vi "fucking PID -- V2.vi"(4 "PID parameters":T4={"I (sec)"=4.747474747474747, "P (sec)"=2.0765656565656565} {"P (sec)" scale=0.01..10.0; "I (sec)" scale=0.01..10.0}, 5 "dt (sec)":dbl=0.02 format="%#_10f", 6 "requested size":i32=100, 7 "PID action":T3, 8 "lorentzian IN":T1={"A (VHz)"=0.003914650866681924, "f (Hz)"=44855.11779996251, "G (Hz)"=2.9247633391664567, "phi(rad)"=3.909694945239435, "Q"=15336.32386569301, "Norm  Ampl"=nan, "bg (V)"=0.00013625172364348747-0.00019483842623467182i, "4corners"={"z (-pi/2)"=-0.0017563199699203156-0.00016210148449623068i, "z(inf)"=0.00013625172364348747-0.00019483842623467182i, "z (pi/2)"=0.0001689886653819286+0.0016977332673291314i, "z center"=-0.0007936656522691936+0.0007678158914164503i, "z(0)"=-0.0017235830281818747+0.0017304702090675725i, "radius"=0.0013384504702515796}} {"bg (V)" format="%#9_9f"; "Q" format="%#9_9f"; "phi(rad)" format="%#9_9f"; "G (Hz)" format="%#9_9f"; "f (Hz)" format="%#9_9f"}, 9 "voltage IN (V)":cdb=-0.0017981943418797428+0.0018232090265536353i format="%#_10f", 10 "time in (sec)":dbl=289.5873590533738, 11 "frequency IN (Hz)":dbl=-1.0 format="%#_10f") -> (0 "lorentzian  OUT":T1={"A (VHz)"=0.003914650866681924, "f (Hz)"=44855.11779996251, "G (Hz)"=2.9247633391664567, "phi(rad)"=3.909694945239435, "Q"=15336.32386569301, "Norm  Ampl"=nan, "bg (V)"=0.00013625172364348747-0.00019483842623467182i, "4corners"={"z (-pi/2)"=-0.0017563199699203156-0.00016210148449623068i, "z(inf)"=0.00013625172364348747-0.00019483842623467182i, "z (pi/2)"=0.0001689886653819286+0.0016977332673291314i, "z center"=-0.0007936656522691936+0.0007678158914164503i, "z(0)"=-0.0017235830281818747+0.0017304702090675725i, "radius"=0.0013384504702515796}} {"bg (V)" format="%#9_9f"; "Q" format="%#9_9f"; "phi(rad)" format="%#9_9f"; "G (Hz)" format="%#9_9f"; "f (Hz)" format="%#9_9f"}, 1 "v out":cdb[](array[numeric])=[-0.0018053953555071376+0.0018127409643177864i, -0.0018165156864968339+0.0018204053176322792i, -0.0017958469040712344+0.0018145950406335631i, -0.0018064864381374278+0.0018213989217676742i, -0.0018205836366976798+0.00181272131689436i, -0.0018068178418151558+0.0017978835138220595i, -0.0018112783584959197+0.0018131542902720791i, -0.001807623114856623+0.0018046251165330447i, -0.0018075769227948962+0.0018141191203122954i, -0.0018125924903436626+0.0018202640246869958i, -0.001797369769488581+0.0018281041177512854i, -0.001810807154127472+0.0018140671984214422i, -0.001801872080007094+0.0018103692059728753i, -0.0018200170226418007+0.0018069703355946354i, -0.0018044272125189902+0.0018419740527244371i, -0.0018048558055226668+0.0018054627086667766i, -0.0018000345238061355+0.001813547911683154i, -0.00179693547343068+0.001827074795896007i, -0.001816753685034828+0.0018283287859578406i, -0.0018100525624063777+0.0018375740151933535i, -0.0018020903561519347+0.001817810965243257i, -0.0018033487515777204+0.0018322759295837736i, -0.001812579170722185+0.0018085274657471593i, -0.0017986956233886219+0.0018369542975809256i, -0.0018110485423681176+0.0018179706114916812i, -0.001818585714895918+0.0018057011713030798i, -0.001817133445971395+0.0018057844840895796i, -0.001815295477436939+0.0018019924367636457i, -0.0018209260305803716+0.0018169201017635879i, -0.0018044295722803938+0.0018022115018756124i, -0.0018311116336601925+0.0018193183868968638i, -0.0018101122757938476+0.0018192759665263973i, -0.0018085434485789354+0.0018163840717862938i, -0.001811836070789227+0.0018293939486975547i, -0.0018092170283701484+0.0018335734859818993i, -0.0018027628167522247+0.0018175751194074211i, -0.0018166463462358528+0.0018270586309948938i, -0.0018043289950367871+0.0018167107559412144i, -0.0018133661975601213+0.0018067609986972299i, -0.0017964121526070878+0.0018212577751918577i, -0.0018005011585912297+0.0018307733988123496i, -0.0018055089150084513+0.0018207057552428135i, -0.0017933683638453196+0.0018290393276094053i, -0.0017947337607063093+0.0018293596839623776i, -0.0018050366985486908+0.0018131516359867486i, -0.001823410598729327+0.0018322386017997551i, -0.0018213270704244217+0.0018092401922307647i, -0.0018195368344010806+0.0018317652375891755i, -0.0018122690298869983+0.0018107874585092214i, -0.0018117815927876852+0.0018193417970865829i, -0.0018241277734167283+0.0018110267815123905i, -0.0018134767100775348+0.0017996041850788186i, -0.0018085781667024604+0.0018109931540198922i, -0.001812588195649308+0.0018242546775294286i, -0.0018038342733790107+0.001816579416119673i, -0.0018219581923603048+0.0018186401375626616i, -0.0018082074467579577+0.0018250013278144528i, -0.0018010302913536497+0.0018340252731910817i, -0.0018095892512791758+0.0018082746963879737i, -0.001806173137863751+0.0018278464093150928i, -0.001806209423211567+0.0018248931786284301i, -0.0018050281395048705+0.0018214527143317128i, -0.001813147159223057+0.0018166873546764629i, -0.0018195040297905845+0.0018213362095911285i, -0.0018038880195332188+0.0018363883332626796i, -0.001811734461819379+0.0018334572150754632i, -0.0018197474636337785+0.001827200887836666i, -0.0017993690496703942+0.0018175740841111926i, -0.0018013879772756337+0.0018034726194164816i, -0.0018044338062849698+0.0018054946939652574i, -0.0018069258232117898+0.001804782758233771i, -0.0018053566300732108+0.001813146961088779i, -0.0018108387556523507+0.0018223068444301986i, -0.0018055103162283466+0.0018170190046832937i, -0.001796024867922929+0.0018240437769777192i, -0.00181063889885541+0.0018058095935931078i, -0.001816760169916204+0.0018115543327705717i, -0.001821094189462785+0.0018078193998815753i, -0.0018114690511362443+0.0018162294699294935i, -0.0018205201141340865+0.001815460678585127i, -0.0017960813076323245+0.0018219635616207451i, -0.0018133234755257535+0.001825049411969287i, -0.001793713870756671+0.001828469705839483i, -0.0018197224487349053+0.001820094212900604i, -0.0018034364661581844+0.0018195335089581947i, -0.0018117189448709056+0.0018188356639653775i, -0.0018008807106835575+0.0018082984011016196i, -0.001802397549962857+0.0018234420699496804i, -0.0018020531158325977+0.0018153058250442436i, -0.0018119913919984066+0.0018153898036333176i, -0.0018073563404384567+0.001819477319147889i, -0.0018121809440278865+0.0018111441608997885i, -0.0018242548595987654+0.0018095956861807342i, -0.0018181047305480982+0.0018060237749628657i, -0.0018154249912101326+0.001810587721306845i, -0.0018155727208419678+0.0018124932447052052i, -0.0018045211817166694+0.0018251170721478073i, -0.0017910521384331079+0.0018331825634809928i, -0.0018064879357469722+0.00182378857110241i, -0.0017981943418797428+0.0018232090265536353i], 2 "freq out":dbl[](array[numeric])=[44853.954031385074, 44853.95417850819, 44853.95416410566, 44853.95436984526, 44853.954673103784, 44853.95452102071, 44853.95394456051, 44853.95323936248, 44853.95230715085, 44853.95139559195, 44853.95052494639, 44853.95024214874, 44853.94983252503, 44853.949439049786, 44853.94854203172, 44853.94838555576, 44853.948031097505, 44853.94780607535, 44853.94808777986, 44853.9483726385, 44853.94903629037, 44853.9497722594, 44853.950879112366, 44853.9515405353, 44853.9528019089, 44853.9538597573, 44853.95426613575, 44853.95412636491, 44853.95345285364, 44853.952516460304, 44853.95139778942, 44853.94987487855, 44853.948493955875, 44853.94721042105, 44853.94623774795, 44853.94570350666, 44853.94534559761, 44853.94503106676, 44853.94481159447, 44853.94422572135, 44853.94406163855, 44853.94439703849, 44853.94482391797, 44853.94582142724, 44853.94730382804, 44853.948592177054, 44853.94970877772, 44853.95018506272, 44853.95065691107, 44853.95081055912, 44853.95089133452, 44853.95041517962, 44853.94942821411, 44853.948370230835, 44853.94746170018, 44853.946719537955, 44853.945737128226, 44853.94501943662, 44853.944922088354, 44853.94457202579, 44853.94453569174, 44853.94471054988, 44853.94502285759, 44853.94515064288, 44853.94506873293, 44853.94552585551, 44853.94620773221, 44853.94675248255, 44853.94744256621, 44853.94788303192, 44853.94807376572, 44853.94796538342, 44853.94782032052, 44853.94772674184, 44853.94768361845, 44853.94807950944, 44853.94808782982, 44853.94773645385, 44853.9468712699, 44853.94597506698, 44853.94481511086, 44853.94416172561, 44853.94361605697, 44853.94372148111, 44853.943585372836, 44853.943613136726, 44853.94357093545, 44853.943481781476, 44853.94366789763, 44853.94391882446, 44853.94398923662, 44853.944105616014, 44853.943951605856, 44853.943228697484, 44853.94206051962, 44853.94066552022, 44853.93910863893, 44853.93796875516, 44853.93771672214, 44853.93766607227], 3 "frequency out (Hz)":dbl=44853.937983312026 format="%#_10f")   [LabVIEW 2018]
uses:
  pid -- parameters.ctl
  PID action.ctl
  lorentzian.ctl
  circle corners.ctl
  four-corner circle transformation.ctl
  agregator -- action.ctl
  linear interpolation iiii- complex.vi
  linear interpolation - real.vi
  Q - not nan -- real.vi
panel:
  out "Plot: complex plane":cluster{dbl[], dbl[]}[](graph)=[{[], []}, {[nan, nan, nan, nan, nan, nan, nan, nan, nan, nan, nan, nan, nan, nan, nan, nan, nan, nan, nan, nan, nan, nan, nan, nan, nan, nan, nan, nan, nan, nan, nan, nan, nan, nan, nan, nan, nan, nan, nan, nan, nan, nan, nan, nan, nan, nan, nan, nan, nan, nan], [nan, nan, nan, nan, nan, nan, nan, nan, nan, nan, nan, nan, nan, nan, nan, nan, nan, nan, nan, nan, nan, nan, nan, nan, nan, nan, nan, nan, nan, nan, nan, nan, nan, nan, nan, nan, nan, nan, nan, nan, nan, nan, nan, nan, nan, nan, nan, nan, nan, nan]}, {[nan, nan, nan, nan, nan, nan, nan, nan, nan, nan, nan, nan, nan, nan, nan, nan, nan, nan, nan, nan], [nan, nan, nan, nan, nan, nan, nan, nan, nan, nan, nan, nan, nan, nan, nan, nan, nan, nan, nan, nan]}, {[nan, nan, nan, nan, nan, nan, nan, nan, nan, nan, nan, nan, nan, nan, nan, nan, nan, nan, nan, nan], [nan, nan, nan, nan, nan, nan, nan, nan, nan, nan, nan, nan, nan, nan, nan, nan, nan, nan, nan, nan]}, {[nan, nan, nan, nan, nan, nan, nan, nan, nan, nan, nan, nan, nan, nan, nan, nan, nan, nan, nan, nan], [nan, nan, nan, nan, nan, nan, nan, nan, nan, nan, nan, nan, nan, nan, nan, nan, nan, nan, nan, nan]}, {[nan, nan, nan, nan, nan, nan, nan, nan, nan, nan, nan, nan, nan, nan, nan, nan, nan, nan, nan, nan], [nan, nan, nan, nan, nan, nan, nan, nan, nan, nan, nan, nan, nan, nan, nan, nan, nan, nan, nan, nan]}, {[], []}]
  in  "Plot: complex plane - filter":cluster{dbl[], dbl[]}[](graph)=[{[], []}, {[], []}, {[0.0, 0.0, 0.0, 0.0, 0.0, 0.0, 0.0, 0.0, 0.0, 0.0, 0.0, 0.0, 0.0, 0.0, 0.0, 0.0, 0.0, 0.0, 0.0, 0.0, 0.0, 0.0, 0.0, 0.0, 0.0, 0.0, 0.0, 0.0, 0.0, 0.0, 0.0, 0.0, 0.0, 0.0, 0.0, 0.0, 0.0, 0.0, 0.0, 0.0, 0.0, 0.0, 0.0, 0.0, 0.0, 0.0, 0.0, 0.0, 0.0, 0.0, 0.0, 0.0, 0.0, 0.0, 0.0, 0.0, 0.0, 0.0, 0.0, 0.0, 0.0, 0.0, 0.0, 0.0, 0.0, 0.0, 0.0, 0.0, 0.0, 0.0, 0.0, 0.0, 0.0, 0.0, 0.0, 0.0, 0.0, 0.0, 0.0, 0.0, 0.0, 0.0, 0.0, 0.0, 0.0, 0.0, 0.0, 0.0, 0.0, 0.0, 0.0, 0.0, 0.0, 0.0, 0.0, 0.0, 0.0, 0.0, 0.0, 0.0], [0.0, 0.0, 0.0, 0.0, 0.0, 0.0, 0.0, 0.0, 0.0, 0.0, 0.0, 0.0, 0.0, 0.0, 0.0, 0.0, 0.0, 0.0, 0.0, 0.0, 0.0, 0.0, 0.0, 0.0, 0.0, 0.0, 0.0, 0.0, 0.0, 0.0, 0.0, 0.0, 0.0, 0.0, 0.0, 0.0, 0.0, 0.0, 0.0, 0.0, 0.0, 0.0, 0.0, 0.0, 0.0, 0.0, 0.0, 0.0, 0.0, 0.0, 0.0, 0.0, 0.0, 0.0, 0.0, 0.0, 0.0, 0.0, 0.0, 0.0, 0.0, 0.0, 0.0, 0.0, 0.0, 0.0, 0.0, 0.0, 0.0, 0.0, 0.0, 0.0, 0.0, 0.0, 0.0, 0.0, 0.0, 0.0, 0.0, 0.0, 0.0, 0.0, 0.0, 0.0, 0.0, 0.0, 0.0, 0.0, 0.0, 0.0, 0.0, 0.0, 0.0, 0.0, 0.0, 0.0, 0.0, 0.0, 0.0, 0.0]}, {[0.0, 0.0, 0.0], [0.0, 0.0, 0.0]}, {[nan, nan, nan, nan, nan, nan, nan, nan, nan, nan, nan, nan, nan, nan, nan, nan, nan, nan, nan, nan], [nan, nan, nan, nan, nan, nan, nan, nan, nan, nan, nan, nan, nan, nan, nan, nan, nan, nan, nan, nan]}, {[0.0, 0.0, 0.0, 0.0, 0.0, 0.0, 0.0, 0.0, 0.0, 0.0, 0.0, 0.0, 0.0, 0.0, 0.0, 0.0, 0.0, 0.0, 0.0, 0.0], [0.0, 0.0, 0.0, 0.0, 0.0, 0.0, 0.0, 0.0, 0.0, 0.0, 0.0, 0.0, 0.0, 0.0, 0.0, 0.0, 0.0, 0.0, 0.0, 0.0]}]
  out "pm lorentzian":T1={"A (VHz)"=nan, "f (Hz)"=0.0, "G (Hz)"=0.0, "phi(rad)"=nan, "Q"=nan, "Norm  Ampl"=nan, "bg (V)"=nan+nani, "4corners"={"z (-pi/2)"=nan+nani, "z(inf)"=nan+nani, "z (pi/2)"=nan+nani, "z center"=nan+nani, "z(0)"=nan+nani, "radius"=nan}} {"bg (V)" format="%#9_9f"; "Q" format="%#9_9f"; "phi(rad)" format="%#9_9f"; "G (Hz)" format="%#9_9f"; "f (Hz)" format="%#9_9f"}
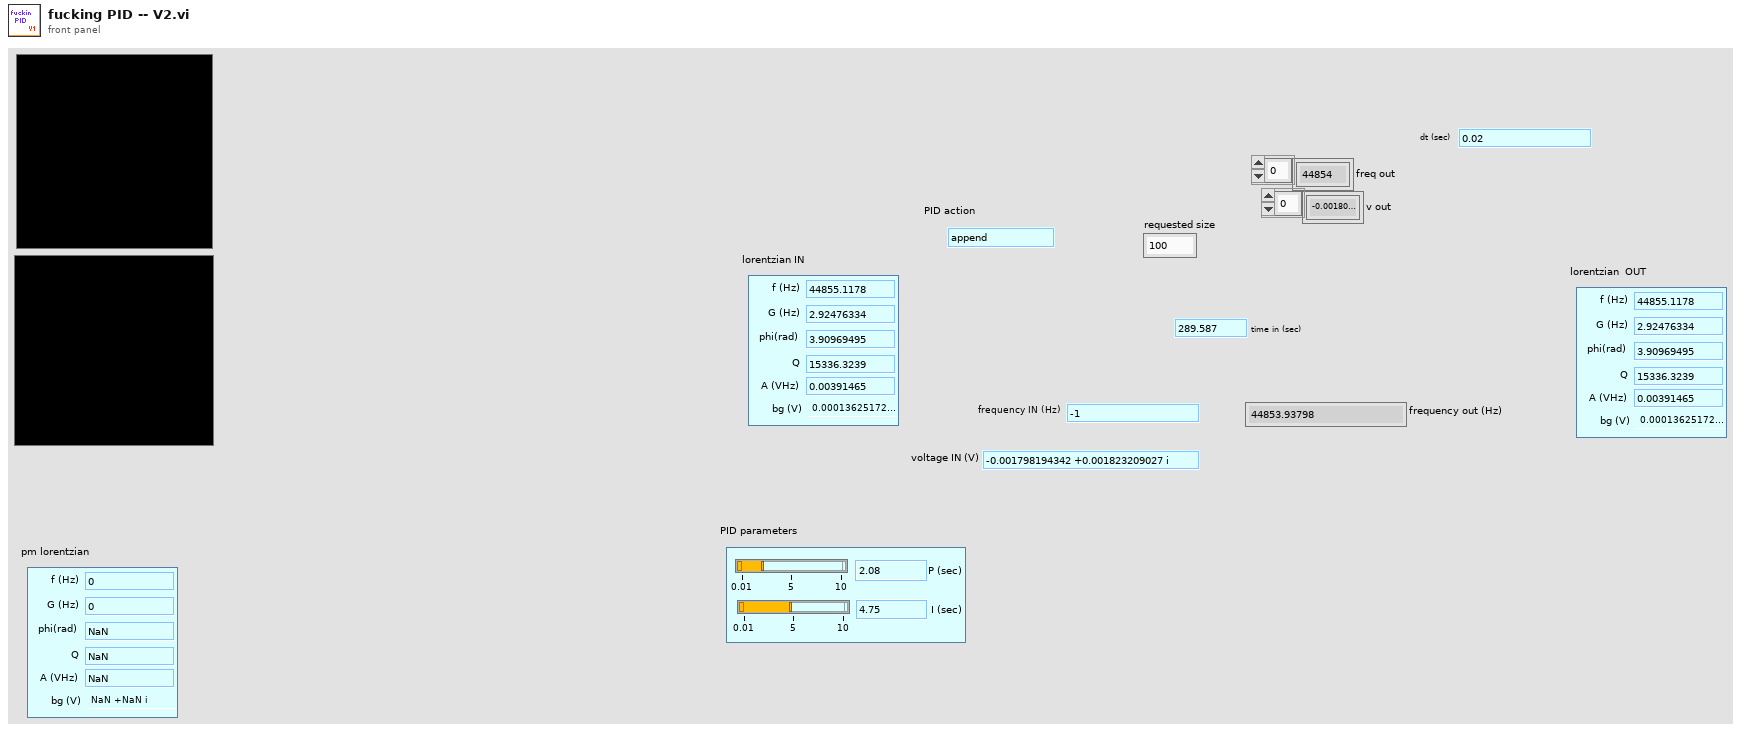
[diagram p1: front panel]
types:
  T1 = typedef "lorentzian.ctl" = cluster{"A (VHz)":dbl, "f (Hz)":dbl, "G (Hz)":dbl, "phi(rad)":dbl, "Q":dbl, "Norm  Ampl":dbl, "bg (V)":cdb, "4corners":T2}
  T2 = typedef "circle corners.ctl" = cluster{"z (-pi/2)":cdb, "z(inf)":cdb, "z (pi/2)":cdb, "z center":cdb, "z(0)":cdb, "radius":dbl}
  T3 = typedef "PID action.ctl" = enum16{"append", "empty!", "reset frequency", "reset from num", "overlimit"}
  T4 = typedef "pid -- parameters.ctl" = cluster{"I (sec)":dbl, "P (sec)":dbl}
  T5 = typedef "four-corner circle transformation.ctl" = enum16{"z(c) z(inf)", "z(c) z(zero)", "fix phase", "calculate lorentzian", "z(0) z(+-pi/2)", "shift to zcenter", "to  canonical", "get canonical phase", "get4corners", "update lorentzian -- from z0", "fake gamma normal", "fake gamma heat", "calculate complex slope"}
  T6 = typedef "agregator -- action.ctl" = enum16{"append", "interpolate", "empty!", "force", "init", "scale", "read last"}
  T7 = typedef "interpolation state - real.ctl" = cluster{"requested size":i32, "Array":dbl[], "actual number of elements":i32}
  T8 = typedef "interpolation state - complex.ctl" = cluster{"requested size":i32, "Array":cdb[], "actual number of elements":i32}
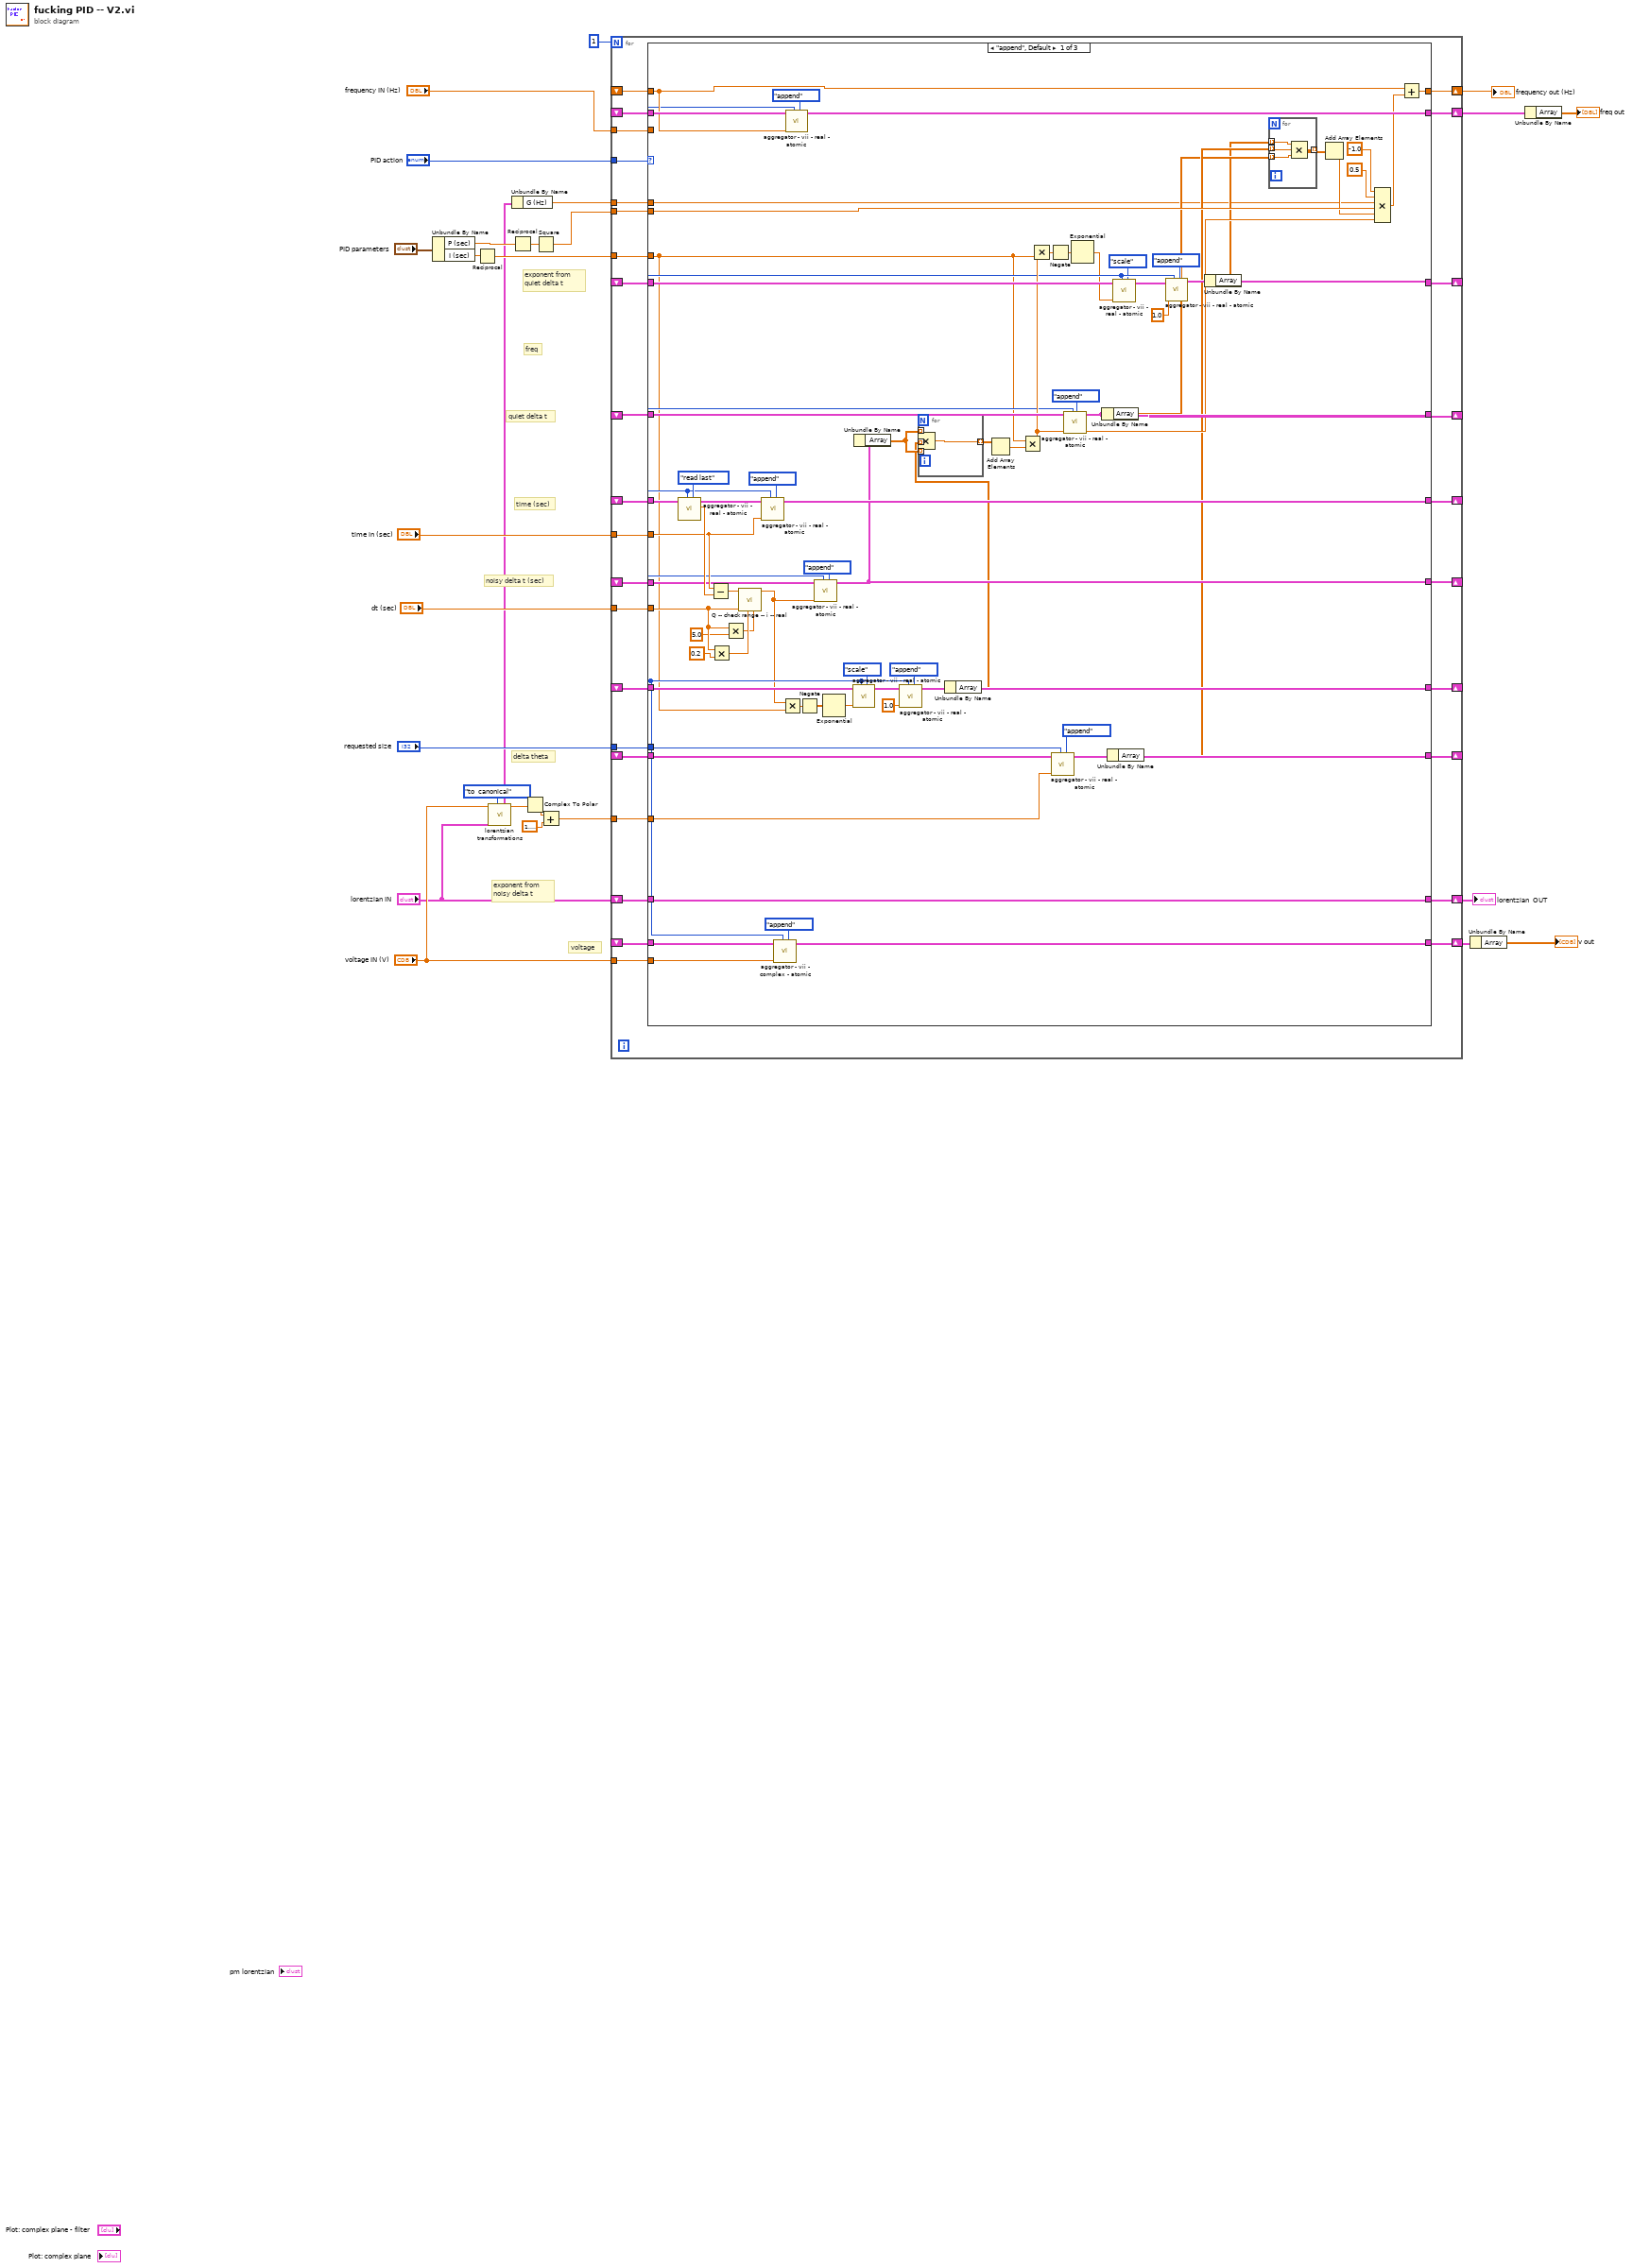
[diagram p0: block diagram]
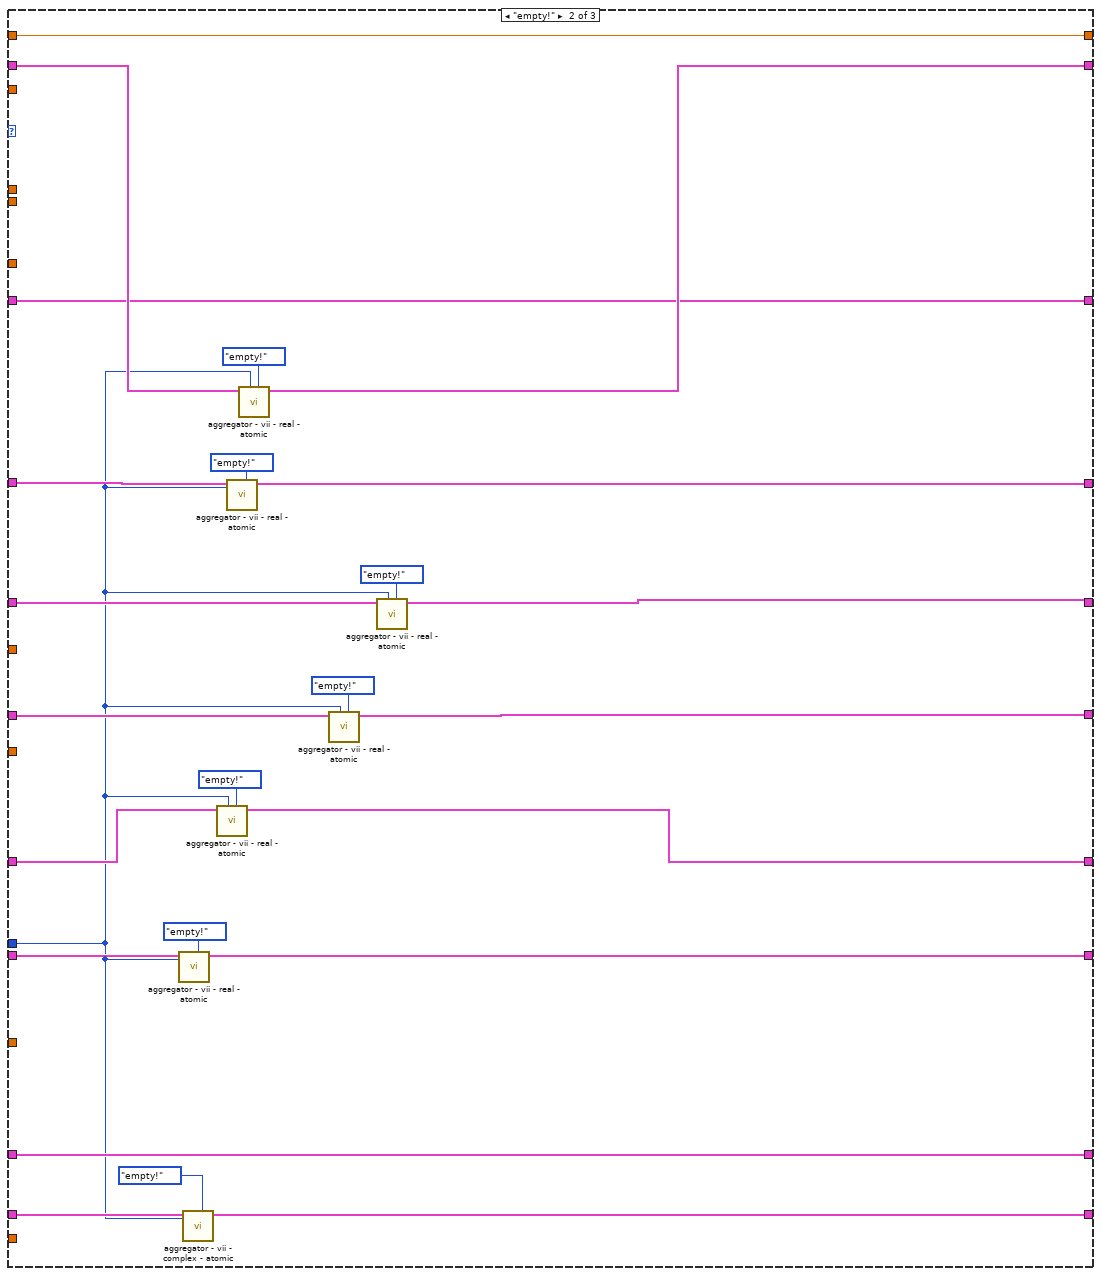
[diagram p2: hidden frame]
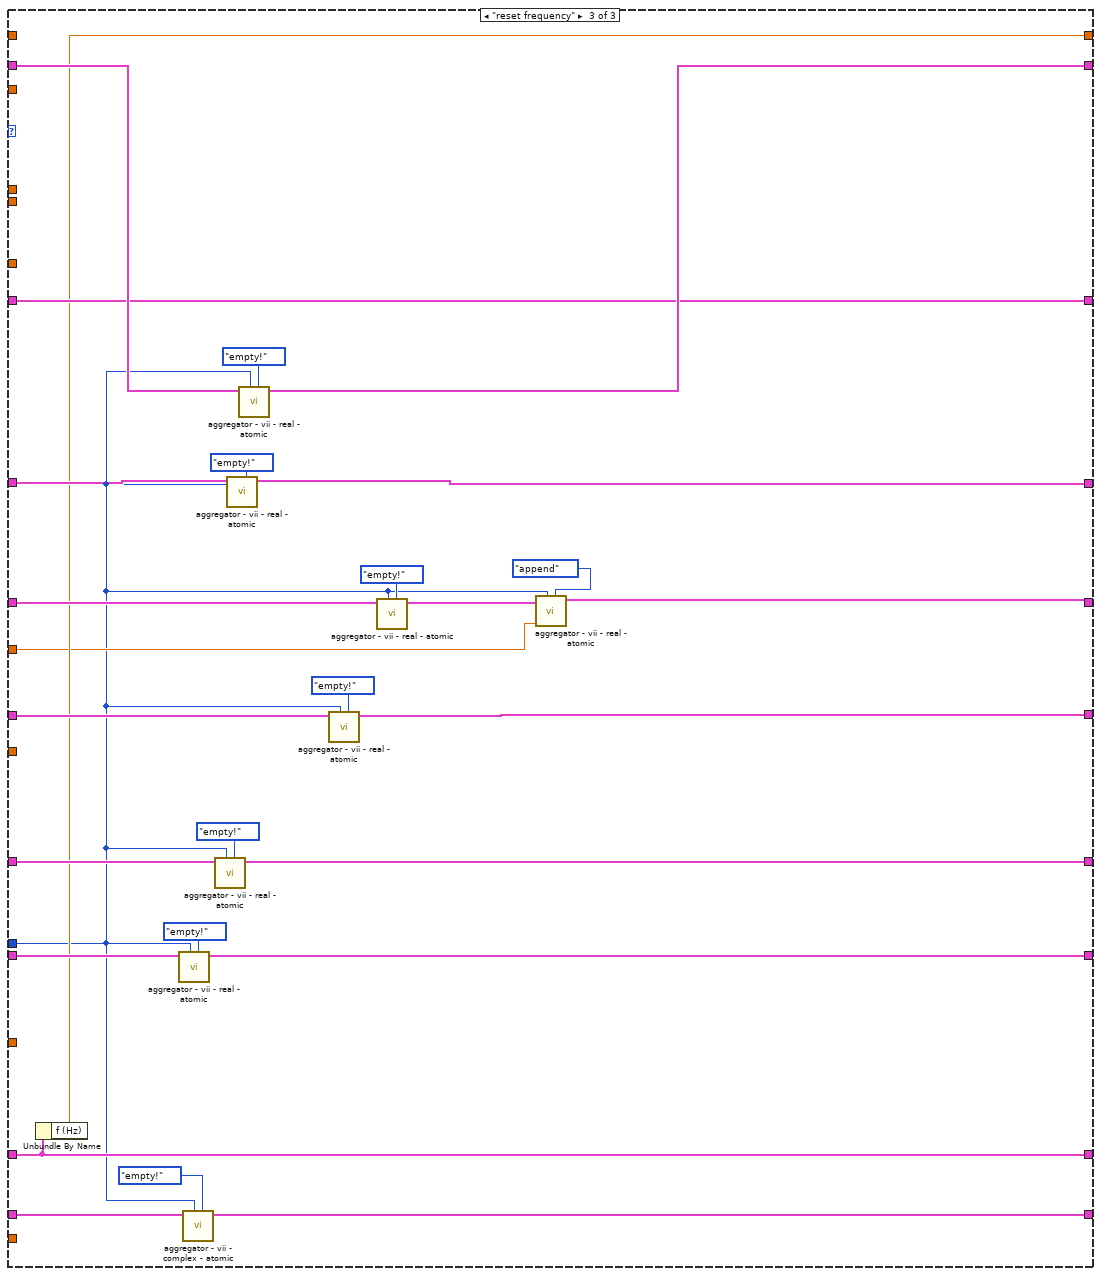
[diagram p3: hidden frame]
diagram:
  # "voltage"
  # "freq"
  # "delta theta"
  # "exponent from \nquiet delta t"
  # "quiet delta t"
  # "time (sec)"
  # "noisy delta t (sec)"
  # "exponent from \nnoisy delta t"
  n1 = Unbundle By Name("PID parameters") -> ("P (sec)"=w19:dbl, "I (sec)"=w21:dbl)
  n2 = Reciprocal(x=w21) -> (1/x=w20:dbl)
  n3 = call "lorentzian transformations.vi"("4 corner circle transformation"=four-corner_circle_transformation."to  canonical", "lorentzian in"="lorentzian IN", "voltage in"="voltage IN (V)") -> ("voltage out"=w7:cdb)  [unwired: 5 in, 3 out]
  n4 = Unbundle By Name("lorentzian IN") -> ("G (Hz)"=w2:dbl)
  n5 = Reciprocal(x=w19) -> (1/x=w18:dbl)
  n6 = Complex To Polar(r * e^(i*theta)=w7) -> (theta=w8:dbl)  [unwired: 1 out]
  n7 = Square(x=w18) -> (x^2=w17:dbl)
  n8 = Add(x=w8, y=1.5707963267948966) -> (x+y=w3:dbl)
  n9 = for {
    N: 1 -> [_]
    tunnel: "requested size" -> [w56]
    tunnel: "PID action" -> [w55]
    shift-right: [w53] -> _
    shift-left: _ -> [w54]
    tunnel: "time in (sec)" -> [w52]
    shift-right: [w50] -> _
    shift-left: _ -> [w51]
    tunnel: w20 -> [w49]
    tunnel: "voltage IN (V)" -> [w48]
    shift-right: [w46] -> _
    shift-left: _ -> [w47]
    shift-right: [w44] -> _
    shift-left: _ -> [w45]
    tunnel: w17 -> [w42]
    shift-right: [w41] -> w16
    shift-left: _ -> [w43]
    shift-right: [w40] -> w15
    shift-left: "lorentzian IN" -> [w39]
    shift-right: [w38] -> w12
    shift-left: _ -> [w37]
    shift-right: [w36] -> w14
    shift-left: _ -> [w35]
    shift-right: [w34] -> _
    shift-left: _ -> [w33]
    shift-right: [w32] -> _
    shift-left: _ -> [w31]
    tunnel: "frequency IN (Hz)" -> [w30]
    tunnel: "dt (sec)" -> [w29]
    tunnel: w3 -> [w28]
    tunnel: w2 -> [w27]
    n10 = case shown="\"append\", Default" w55 {
      tunnel: w56 -> [w83 w135 w159]
      tunnel: w54 -> [w125 w148 w176]
      tunnel: [w105 w134 w161] -> w53
      tunnel: w52 -> [w116 _ w160]
      tunnel: w51 -> [w124 w152 w180]
      tunnel: [w110 w151 w179] -> w50
      tunnel: w49 -> [w62 _ _]
      tunnel: w48 -> [w99 _ _]
      tunnel: w47 -> [w91 w150 w178]
      tunnel: [w78 w149 w177] -> w46
      tunnel: w45 -> [w114 w154 w182]
      tunnel: [w112 w153 w181] -> w44
      tunnel: w43 -> [w96 w147 _]
      tunnel: w39 -> [w102 w146 w165]
      tunnel: w42 -> [w109 _ _]
      tunnel: [w107 w147 w164] -> w41
      tunnel: [w102 w146 w165] -> w40
      tunnel: [w101 w144 w174] -> w38
      tunnel: w37 -> [w100 w145 w175]
      tunnel: [w98 w140 w170] -> w36
      tunnel: w35 -> [w97 w141 w171]
      tunnel: [w80 w138 w168] -> w34
      tunnel: w33 -> [w88 w137 w167]
      tunnel: [w79 w136 w166] -> w32
      tunnel: w31 -> [w87 w136 w166]
      tunnel: w30 -> [_ _ _]
      tunnel: w29 -> [w63 _ _]
      tunnel: w28 -> [w58 _ _]
      tunnel: w27 -> [w57 _ _]
      frame "append", Default {
        n11 = call "aggregator - vii - real - atomic.vi"("aggregator action"=agregator_--_action."read last", "requested size"=w83, "state IN"=w125) -> ("mean"=w118:dbl, "state OUT"=w106:T7)  [unwired: 5 in, 2 out]
        n12 = Subtract(x=w116, y=w118) -> (x-y=w73:dbl)
        n13 = Multiply(x=w63, y=0.2 ("upper")) -> (x*y=w69:dbl)
        n14 = Multiply(x=w63, y=5.0 ("upper")) -> (x*y=w60:dbl)
        n15 = call "Q -- check range -- i -- real.vi"("upper"=w60, "lower"=w69, "default"=w63, "number"=w73) -> ("number in range"=w71:dbl)  [unwired: 5 in, 2 out]
        n16 = call "aggregator - vii - real - atomic.vi"("aggregator action"=agregator_--_action."append", "requested size"=w83, "number"=w116, "state IN"=w106) -> ("state OUT"=w105:T7)  [unwired: 4 in, 3 out]
        n17 = call "aggregator - vii - complex - atomic.vi"("aggregator action"=agregator_--_action."append", "requested size"=w83, "number"=w99, "state IN"=w100) -> ("state OUT"=w101:T8)  [unwired: 4 in, 3 out]
        n18 = Multiply(x=w71, y=w62) -> (x*y=w75:dbl)
        n19 = call "aggregator - vii - real - atomic.vi"("aggregator action"=agregator_--_action."append", "requested size"=w83, "number"=w96, "state IN"=w97) -> ("state OUT"=w98:T7)  [unwired: 4 in, 3 out]
        n20 = Negate(x=w75) -> (-x=w72:dbl)
        n21 = call "aggregator - vii - real - atomic.vi"("aggregator action"=agregator_--_action."append", "requested size"=w83, "number"=w71, "state IN"=w91) -> ("state OUT"=w78:T7)  [unwired: 4 in, 3 out]
        n22 = Exponential(1:w72) -> (0:w74:dbl)
        n23 = call "aggregator - vii - real - atomic.vi"("aggregator action"=agregator_--_action."scale", "requested size"=w83, "number"=w74, "state IN"=w124) -> ("state OUT"=w123:T7)  [unwired: 4 in, 3 out]
        n24 = Unbundle By Name(w78) -> ("Array"=w90:dbl[])
        n25 = call "aggregator - vii - real - atomic.vi"("aggregator action"=agregator_--_action."append", "requested size"=w83, "number"=1.0, "state IN"=w123) -> ("state OUT"=w110:T7)  [unwired: 4 in, 3 out]
        n26 = Unbundle By Name(w110) -> ("Array"=w77:dbl[])
        n27 = for {
          tunnel: [w129] -> w92 mode=indexing
          tunnel: w90 -> [w128] mode=indexing
          tunnel: w77 -> [w127] mode=indexing
          tunnel: w90 -> [w126] mode=indexing
          n28 = Compound Arithmetic op=MULTIPLY(w128, w127, w126) -> (w129:dbl)
        }
        n29 = Add Array Elements(numeric array=w92) -> (sum=w61:dbl)
        n30 = Multiply(x=w62, y=w61) -> (x*y=w86:dbl)
        n31 = Multiply(x=w86, y=w62) -> (x*y=w66:dbl)
        n32 = Negate(x=w66) -> (-x=w65:dbl)
        n33 = call "aggregator - vii - real - atomic.vi"("aggregator action"=agregator_--_action."append", "requested size"=w83, "number"=w58, "state IN"=w114) -> ("state OUT"=w112:T7)  [unwired: 4 in, 3 out]
        n34 = call "aggregator - vii - real - atomic.vi"("aggregator action"=agregator_--_action."append", "requested size"=w83, "number"=w86, "state IN"=w88) -> ("state OUT"=w80:T7)  [unwired: 4 in, 3 out]
        n35 = Exponential(1:w65) -> (0:w64:dbl)
        n36 = Unbundle By Name(w80) -> ("Array"=w68:dbl[])
        n37 = Unbundle By Name(w112) -> ("Array"=w76:dbl[])
        n38 = call "aggregator - vii - real - atomic.vi"("aggregator action"=agregator_--_action."scale", "requested size"=w83, "number"=w64, "state IN"=w87) -> ("state OUT"=w85:T7)  [unwired: 4 in, 3 out]
        n39 = call "aggregator - vii - real - atomic.vi"("aggregator action"=agregator_--_action."append", "requested size"=w83, "number"=1.0, "state IN"=w85) -> ("state OUT"=w79:T7)  [unwired: 4 in, 3 out]
        n40 = Unbundle By Name(w79) -> ("Array"=w67:dbl[])
        n41 = for {
          tunnel: w76 -> [w133] mode=indexing
          tunnel: [w132] -> w111 mode=indexing
          tunnel: w68 -> [w131] mode=indexing
          tunnel: w67 -> [w130] mode=indexing
          n42 = Compound Arithmetic op=MULTIPLY(w130, w133, w131) -> (w132:dbl)
        }
        n43 = Add Array Elements(numeric array=w111) -> (sum=w108:dbl)
        n44 = Compound Arithmetic op=MULTIPLY(-1.0 ("value"), 0.5 ("value"), w57, w109, w108, w86) -> (w93:dbl)
        n45 = Add(x=w96, y=w93) -> (x+y=w107:dbl)
      }
      frame "empty!" {
        n46 = call "aggregator - vii - real - atomic.vi"("aggregator action"=agregator_--_action."empty!", "requested size"=w135, "state IN"=w154) -> ("state OUT"=w153:T7)  [unwired: 5 in, 3 out]
        n47 = call "aggregator - vii - complex - atomic.vi"("aggregator action"=agregator_--_action."empty!", "requested size"=w135, "state IN"=w145) -> ("state OUT"=w144:T8)  [unwired: 5 in, 3 out]
        n48 = call "aggregator - vii - real - atomic.vi"("aggregator action"=agregator_--_action."empty!", "requested size"=w135, "state IN"=w152) -> ("state OUT"=w151:T7)  [unwired: 5 in, 3 out]
        n49 = call "aggregator - vii - real - atomic.vi"("aggregator action"=agregator_--_action."empty!", "requested size"=w135, "state IN"=w137) -> ("state OUT"=w138:T7)  [unwired: 5 in, 3 out]
        n50 = call "aggregator - vii - real - atomic.vi"("aggregator action"=agregator_--_action."empty!", "requested size"=w135, "state IN"=w141) -> ("state OUT"=w140:T7)  [unwired: 5 in, 3 out]
        n51 = call "aggregator - vii - real - atomic.vi"("aggregator action"=agregator_--_action."empty!", "requested size"=w135, "state IN"=w150) -> ("state OUT"=w149:T7)  [unwired: 5 in, 3 out]
        n52 = call "aggregator - vii - real - atomic.vi"("aggregator action"=agregator_--_action."empty!", "requested size"=w135, "state IN"=w148) -> ("state OUT"=w134:T7)  [unwired: 5 in, 3 out]
      }
      frame "reset frequency" {
        n53 = Unbundle By Name(w165) -> ("f (Hz)"=w164:dbl)
        n54 = call "aggregator - vii - real - atomic.vi"("aggregator action"=agregator_--_action."empty!", "requested size"=w159, "state IN"=w182) -> ("state OUT"=w181:T7)  [unwired: 5 in, 3 out]
        n55 = call "aggregator - vii - complex - atomic.vi"("aggregator action"=agregator_--_action."empty!", "requested size"=w159, "state IN"=w175) -> ("state OUT"=w174:T8)  [unwired: 5 in, 3 out]
        n56 = call "aggregator - vii - real - atomic.vi"("aggregator action"=agregator_--_action."empty!", "requested size"=w159, "state IN"=w180) -> ("state OUT"=w179:T7)  [unwired: 5 in, 3 out]
        n57 = call "aggregator - vii - real - atomic.vi"("aggregator action"=agregator_--_action."empty!", "requested size"=w159, "state IN"=w167) -> ("state OUT"=w168:T7)  [unwired: 5 in, 3 out]
        n58 = call "aggregator - vii - real - atomic.vi"("aggregator action"=agregator_--_action."empty!", "requested size"=w159, "state IN"=w171) -> ("state OUT"=w170:T7)  [unwired: 5 in, 3 out]
        n59 = call "aggregator - vii - real - atomic.vi"("aggregator action"=agregator_--_action."empty!", "requested size"=w159, "state IN"=w178) -> ("state OUT"=w177:T7)  [unwired: 5 in, 3 out]
        n60 = call "aggregator - vii - real - atomic.vi"("aggregator action"=agregator_--_action."empty!", "requested size"=w159, "state IN"=w176) -> ("state OUT"=w162:T7)  [unwired: 5 in, 3 out]
        n61 = call "aggregator - vii - real - atomic.vi"("aggregator action"=agregator_--_action."append", "requested size"=w159, "number"=w160, "state IN"=w162) -> ("state OUT"=w161:T7)  [unwired: 4 in, 3 out]
      }
    }
  }
  "frequency out (Hz)" <- w16
  "lorentzian  OUT" <- w15
  n62 = Unbundle By Name(w12) -> ("Array"=→"v out":cdb[])
  n63 = Unbundle By Name(w14) -> ("Array"=→"freq out":dbl[])
